vi "백업serial del.vi"() -> ()   [LabVIEW 2014]
uses:
  <vilib>/Utility/sysdir.llb/System Directory Type.ctl
panel:
  in  "정규식":string
  in  "정규식 2":string
types:
  T1 = enum16{"open", "replace", "create", "open or create", "replace or create", "replace or create with confirmation"}
  T2 = typedef "System Directory Type.ctl" = i32
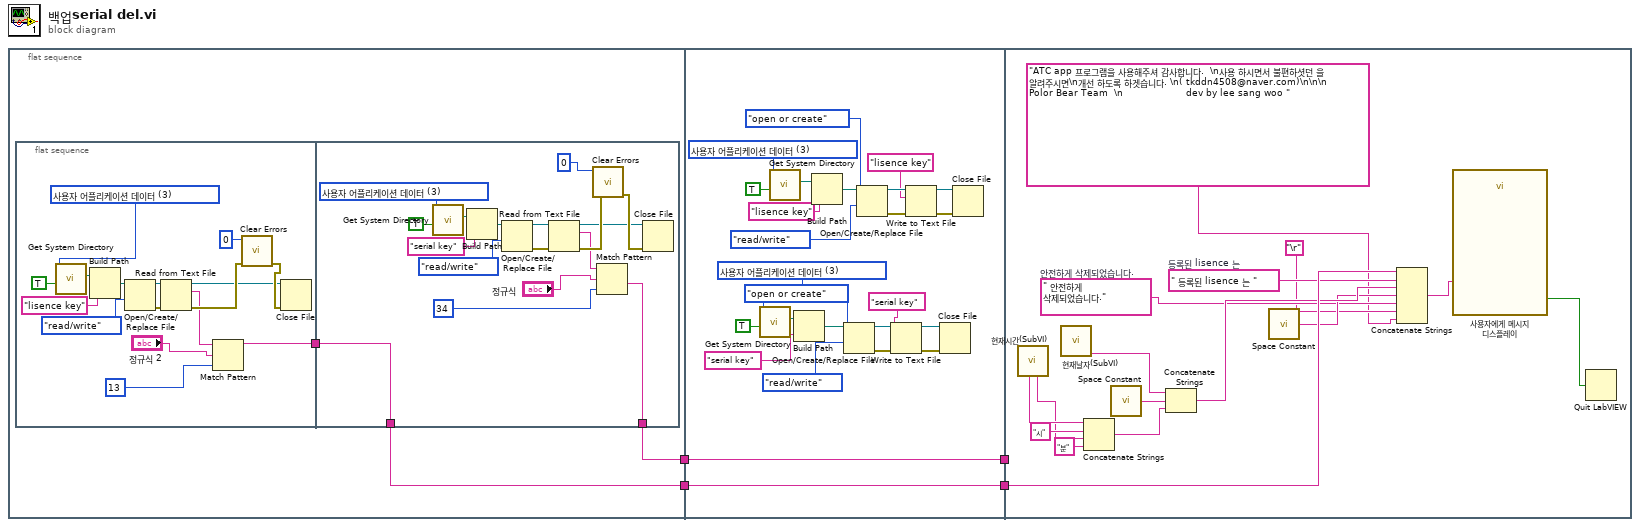
[diagram p0: block diagram]
diagram:
  n1 = flat-sequence {
    tunnel: [w6] -> w4
    tunnel: [w5] -> w2
    tunnel: w4 -> [w41]
    tunnel: [w42] -> w3
    tunnel: w2 -> [w42]
    tunnel: [w41] -> w1
    tunnel: w3 -> [w82]
    tunnel: w1 -> [_]
    frame #0 {
      n2 = flat-sequence {
        tunnel: [w8] -> w7
        tunnel: w7 -> [w24]
        tunnel: [w25] -> w6
        tunnel: [w24] -> w5
        frame #0 {
          w13 = T2 3 items=["사용자 홈"=0, "사용자 데스크탑"=1, "사용자 문서"=2, "사용자 어플리케이션 데이터"=3, "사용자 환경"=4, "사용자 임시"=5, "퍼블릭 문서"=6, "퍼블릭 어플리케이션 데이터"=7, "퍼블릭 환경"=8, "퍼블릭 캐시"=13, "시스템 코어 라이브러리"=9, "시스템 설치된 라이브러리"=10, "어플리케이션 파일"=11, "부팅 볼륨 루트"=12] ("system directory type")
          n3 = call <vilib>:"Get System Directory.vi"("create directory if not found? (F)"=TRUE, "system directory type"=w13) -> ("system directory"=w12:path)  [unwired: 9 in]
          n4 = Build Path(base path=w12, name or relative path="lisence key" ("이름 또는 상대 경로")) -> (appended path=w11:path)
          n5 = Open/Create/Replace File(file path (use dialog)=w11, access (0:read/write)=enum16{"read/write", "read-only", "write-only"}."read/write" ("접근(0:읽기/쓰기)")) -> (refnum out=w17:refnum<file>, error out=w16:errorcluster)  [unwired: 4 in, 1 out]
          n6 = Read from Text File(file (use dialog)=w17, error in=w16) -> (refnum out=w18:refnum<file>, text=w19:string, error out=w21:errorcluster)  [unwired: 2 in, 1 out]
          n7 = Match Pattern(string=w19, regular expression="정규식 2", offset (0)=13 ("오프셋(0) 2")) -> (before substring=w8:string)  [unwired: 3 out]
          n8 = call <vilib>:"Clear Errors.vi"("error in (no error)"=w21, "specific error code to clear (0: all)"=0) -> ("error out"=w22:errorcluster)  [unwired: 4 in, 1 out]
          n9 = Close File(refnum=w18, error in=w22) -> ()  [unwired: 2 out]
        }
        frame #1 {
          w33 = T2 3 items=["사용자 홈"=0, "사용자 데스크탑"=1, "사용자 문서"=2, "사용자 어플리케이션 데이터"=3, "사용자 환경"=4, "사용자 임시"=5, "퍼블릭 문서"=6, "퍼블릭 어플리케이션 데이터"=7, "퍼블릭 환경"=8, "퍼블릭 캐시"=13, "시스템 코어 라이브러리"=9, "시스템 설치된 라이브러리"=10, "어플리케이션 파일"=11, "부팅 볼륨 루트"=12] ("system directory type")
          n10 = call <vilib>:"Get System Directory.vi"("create directory if not found? (F)"=TRUE, "system directory type"=w33) -> ("system directory"=w34:path)  [unwired: 9 in]
          n11 = Build Path(base path=w34, name or relative path="serial key" ("이름 또는 상대 경로")) -> (appended path=w35:path)
          n12 = Open/Create/Replace File(file path (use dialog)=w35, access (0:read/write)=enum16{"read/write", "read-only", "write-only"}."read/write" ("접근(0:읽기/쓰기)")) -> (refnum out=w29:refnum<file>, error out=w30:errorcluster)  [unwired: 4 in, 1 out]
          n13 = Read from Text File(file (use dialog)=w29, error in=w30) -> (refnum out=w28:refnum<file>, text=w36:string, error out=w38:errorcluster)  [unwired: 2 in, 1 out]
          n14 = call <vilib>:"Clear Errors.vi"("error in (no error)"=w38, "specific error code to clear (0: all)"=0) -> ("error out"=w39:errorcluster)  [unwired: 4 in, 1 out]
          n15 = Match Pattern(string=w36, regular expression="정규식", offset (0)=34 ("오프셋(0)")) -> (after substring=w25:string)  [unwired: 3 out]
          n16 = Close File(refnum=w28, error in=w39) -> ()  [unwired: 2 out]
        }
      }
    }
    frame #1 {
      w50 = T2 3 items=["사용자 홈"=0, "사용자 데스크탑"=1, "사용자 문서"=2, "사용자 어플리케이션 데이터"=3, "사용자 환경"=4, "사용자 임시"=5, "퍼블릭 문서"=6, "퍼블릭 어플리케이션 데이터"=7, "퍼블릭 환경"=8, "퍼블릭 캐시"=13, "시스템 코어 라이브러리"=9, "시스템 설치된 라이브러리"=10, "어플리케이션 파일"=11, "부팅 볼륨 루트"=12] ("system directory type")
      w62 = T2 3 items=["사용자 홈"=0, "사용자 데스크탑"=1, "사용자 문서"=2, "사용자 어플리케이션 데이터"=3, "사용자 환경"=4, "사용자 임시"=5, "퍼블릭 문서"=6, "퍼블릭 어플리케이션 데이터"=7, "퍼블릭 환경"=8, "퍼블릭 캐시"=13, "시스템 코어 라이브러리"=9, "시스템 설치된 라이브러리"=10, "어플리케이션 파일"=11, "부팅 볼륨 루트"=12] ("system directory type")
      n17 = call <vilib>:"Get System Directory.vi"("create directory if not found? (F)"=TRUE, "system directory type"=w62) -> ("system directory"=w63:path)  [unwired: 9 in]
      n18 = call <vilib>:"Get System Directory.vi"("create directory if not found? (F)"=TRUE, "system directory type"=w50) -> ("system directory"=w49:path)  [unwired: 9 in]
      n19 = Build Path(base path=w63, name or relative path="serial key" ("이름 또는 상대 경로")) -> (appended path=w64:path)
      n20 = Build Path(base path=w49, name or relative path="lisence key" ("이름 또는 상대 경로")) -> (appended path=w48:path)
      n21 = Open/Create/Replace File(file path (use dialog)=w64, operation (0:open)=T1."open or create" ("동작(0:open)"), access (0:read/write)=enum16{"read/write", "read-only", "write-only"}."read/write" ("접근(0:읽기/쓰기)")) -> (refnum out=w57:refnum<file>, error out=w58:errorcluster)  [unwired: 3 in, 1 out]
      n22 = Open/Create/Replace File(file path (use dialog)=w48, operation (0:open)=T1."open or create" ("동작(0:open)"), access (0:read/write)=enum16{"read/write", "read-only", "write-only"}."read/write" ("접근(0:읽기/쓰기)")) -> (refnum out=w52:refnum<file>, error out=w53:errorcluster)  [unwired: 3 in, 1 out]
      n23 = Write to Text File(file (use dialog)=w57, text="serial key" ("이름 또는 상대 경로"), error in=w58) -> (refnum out=w60:refnum<file>, error out=w59:errorcluster)  [unwired: 1 in, 1 out]
      n24 = Write to Text File(file (use dialog)=w52, text="lisence key" ("이름 또는 상대 경로"), error in=w53) -> (refnum out=w51:refnum<file>, error out=w54:errorcluster)  [unwired: 1 in, 1 out]
      n25 = Close File(refnum=w60, error in=w59) -> ()  [unwired: 2 out]
      n26 = Close File(refnum=w51, error in=w54) -> ()  [unwired: 2 out]
    }
    frame #2 {
      w73 = " 등록된 lisence 는 "  # 등록된 lisence 는
      w70 = " 안전하게 삭제되었습니다."  # 안전하게 삭제되었습니다.
      n27 = call "현재시간(SubVI).vi"() -> ("분 문자열"=w78:string, "시 문자열"=w80:string)  [unwired: 3 in, 7 out]
      n28 = call "현재날자(SubVI).vi"() -> ("월,일 을 문자열로"=w74:string)  [unwired: 5 in, 6 out]
      n29 = Concatenate Strings(w80, "시", w78, "분" ("문자열")) -> (w76:string)
      n30 = call <vilib>:"Space Constant.vi"() -> ("String"=w75:string)
      n31 = Concatenate Strings(w74, w75, w76) -> (w72:string)
      n32 = call <vilib>:"Space Constant.vi"() -> ("String"=w71:string)
      n33 = Concatenate Strings(w82, w73, w72, w71, w70, "\r", "ATC app 프로그램을 사용해주셔 감사합니다.  \n사용 하시면서 불편하셧던 을 알려주시면\n개선 하도록 하겟습니다. \n( tkddn4508@naver.com)\n\n\n                           Polor Bear Team  \n                     dev by lee sang woo " ("Message")) -> (w81:string)
      n34 = call "사용자에게 메시지 디스플레이"("Message"=w81) -> ("확인"=w67:bool)  [unwired: 9 in, 1 out]
      n35 = Quit LabVIEW(quit? (T)=w67) -> ()
    }
  }
